vi "SetVolumeLabel.vi"(1 "error in (no error)":errorcluster, 2 "VolumeName":string, 3 "RootPathName (C:\\)":string="c:\\") -> (0 "error out":errorcluster)   [LabVIEW 2011]
doc: "Sets the Volume Label string associated with the drive"
uses:
  kernel32.dll
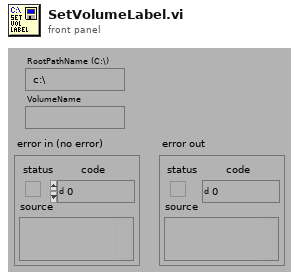
[diagram p1: front panel]
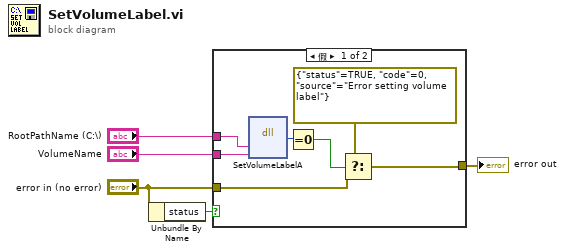
[diagram p0: block diagram]
diagram:
  n1 = Unbundle By Name("error in (no error)") -> ("status"=w1:bool)
  n2 = case shown="假" w1 {
    tunnel: "RootPathName (C:\\)" -> [w12 _]
    tunnel: "VolumeName" -> [w11 _]
    tunnel: "error in (no error)" -> [w8 w13]
    tunnel: [w6 w13] -> w3
    frame False {
      n3 = dll-call lib="kernel32.dll" fn="SetVolumeLabelA" label="Set Volume Label"("lpRootPathName"=w12, "lpVolumeName"=w11) -> (w10:u8)  [unwired: 5 in, 2 out]
      n4 = Equal To 0?(x=w10) -> (x = 0?=w9:bool)
      n5 = Select(t=errorcluster {"status"=TRUE, "code"=0, "source"="Error setting volume label"}, s=w9, f=w8) -> (s? t:f=w6:errorcluster)
    }
    frame True {
      # "NOP"
    }
  }
  "error out" <- w3
